vi "RT_Call Read.vi"(8 "error in":errorcluster, 11 "FPGA VI Reference In":T1) -> (0 "error out":errorcluster, 2 "Data Out":u8, 3 "FPGA VI Reference Out":T1)   [LabVIEW 2018]
uses:
  Data Def/RT_FPGA VI Reference.ctl
  <vilib>/Utility/error.llb/Error Cluster From Error Code.vi
  <vilib>/rvi/errors/niLvFpgaAdjustHostInterfaceError.vi
  <vilib>/rvi/interface/nirviReadWriteControl/nirviReadWriteControl.xnode
  <vilib>/rvi/interface/Simulation/niFpgaSimulationCallBeginRW.vi
  NiFpgaLv.dll
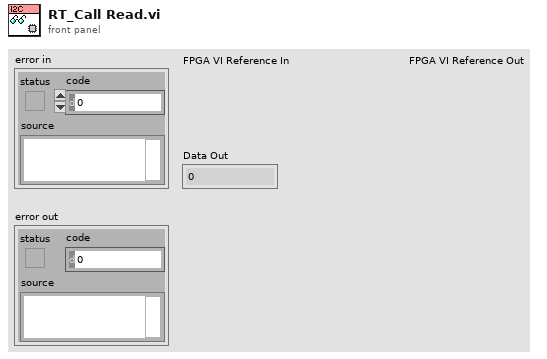
[diagram p1: front panel]
types:
  T1 = typedef "RT_FPGA VI Reference.ctl" = refnum<k20>
  T2 = enum16{"Idle", "Set Idle", "Config", "Read", "Write", "Arm", "Auto Run", "Auto Config", "Auto Write", "Auto Arm", "Auto Read", "Auto Check"}
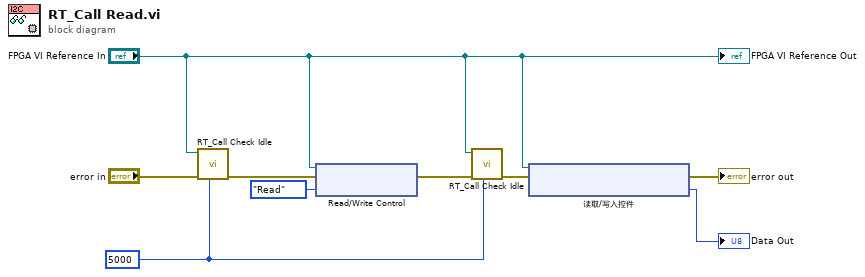
[diagram p0: block diagram]
diagram:
  w6 = 5000 ("Timeout?")
  n1 = call "RT_Call Check Idle.vi"("Timeout?"=w6, "error in"="error in", "FPGA VI Reference In"="FPGA VI Reference In") -> ("error out"=w5:errorcluster)  [unwired: 7 in, 1 out]
  n2 = xnode "Read/Write Control"("FPGA VI Reference In"="FPGA VI Reference In", "error in"=w5, "I2C Loop State"=T2."Read") -> ("error out"=w4:errorcluster)  [unwired: 1 out]
  n3 = call "RT_Call Check Idle.vi"("Timeout?"=w6, "error in"=w4, "FPGA VI Reference In"="FPGA VI Reference In") -> ("error out"=w3:errorcluster)  [unwired: 7 in, 1 out]
  n4 = xnode "读取/写入控件"("FPGA VI Reference In"="FPGA VI Reference In", "error in"=w3) -> ("error out"=→"error out":errorcluster, "I2C Protocol Output Data"=→"Data Out":u8)  [unwired: 1 out]
  "FPGA VI Reference Out" <- "FPGA VI Reference In"
